vi "Parse Number.vi"(10 "String":string) -> (1 "Leading Zero?":bool, 2 "Number":i32)   [LabVIEW 2017, in "Semver.lvlib" / "Semver.lvclass"]
uses:
  Semver.lvclass
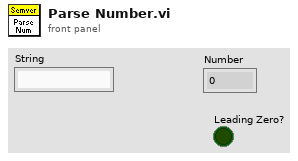
[diagram p1: front panel]
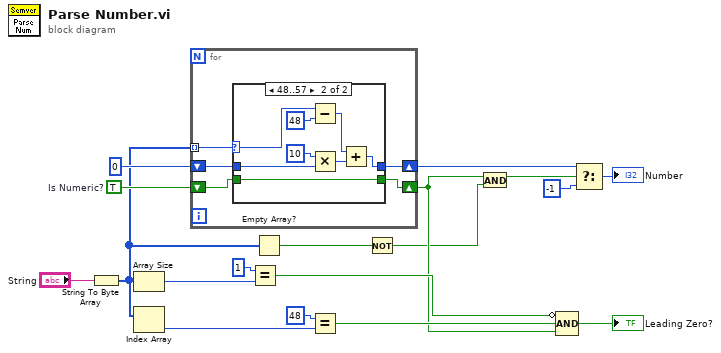
[diagram p0: block diagram]
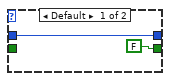
[diagram p2: hidden frame]
diagram:
  w18 = TRUE  # Is Numeric?
  n1 = String To Byte Array(string="String") -> (unsigned byte array=w3:u8[])
  n2 = Array Size(array=w3) -> (size(s)=w13:i32)
  n3 = Index Array(array=w3) -> (element=w16:u8)  [unwired: 1 in]
  n4 = for {
    tunnel: w3 -> [w23] mode=indexing
    shift-right: [w21] -> w8
    shift-left: w18 -> [w22]
    shift-right: [w19] -> w7
    shift-left: 0 -> [w20]
    n5 = case shown="48..57" w23 {
      selector: w23 -> [_ w32]
      tunnel: w22 -> [_ w33]
      tunnel: [FALSE w33] -> w21
      tunnel: w20 -> [w24 w30]
      tunnel: [w24 w27] -> w19
      frame Default {
      }
      frame 48..57 {
        n6 = Subtract(x=w32, y=u8 48) -> (x-y=w26:u8)
        n7 = Multiply(x=10, y=w30) -> (x*y=w29:i32)
        n8 = Add(x=w26, y=w29) -> (x+y=w27:i32)
      }
    }
  }
  n9 = Equal?(x=1, y=w13) -> (x = y?=w11:bool)
  n10 = Empty Array?(array=w3) -> (empty?=w2:bool)
  n11 = Equal?(x=u8 48, y=w16) -> (x = y?=w14:bool)
  n12 = Not(x=w2) -> (.not. x?=w1:bool)
  n13 = And(x=w8, y=w1) -> (x .and. y?=w4:bool)
  n14 = Compound Arithmetic op=AND(invert w11, w14, w8) -> (→"Leading Zero?":bool)
  n15 = Select(t=w7, s=w4, f=-1) -> (s? t:f=→"Number":i32)
